vi "AD5535 Manager.vi"() -> ()   [LabVIEW 2016]
uses:
  Typedef/AD5535 - Multi sweep settings.ctl
  Typedef/AD5535 - Square wave settings.ctl
  Typedef/AD5535 - States.ctl
  Typedef/AD5535 - Sweep settings.ctl
panel:
  in  "Exit":bool
  in  "Tab Control":T1(tab)
  in  "Reset all to 0":bool
  in  "Update all":bool
  in  "Update channel":bool
  in  "Channel":u8 max=31 step=1
  in  "Value":sgl min=0 max=204.8 step=0.0125 format="%#_g V"
  in  "Vstep":sgl=0.0125 min=0.0125 max=204.8 step=0.0125 format="%#_g V"
  in  "Vstop":sgl min=0 max=204.8 step=0.0125 format="%#_g V"
  in  "Vstart":sgl min=0 max=204.8 step=0.0125 format="%#_g V"
  in  "Channel to sweep":u8 max=31 step=1
  in  "All other chans value":sgl min=0 max=204.8 step=0.0125 format="%#_g V"
  in  "Time interval - Single sweep":u32=10 caption="Time interval" min=10 max=20000 step=5 format="%.0f ms"
  in  "Sweep channel":bool
  in  "Multi-sweep settings":T2 {"Vstep" min=0.0125 max=204.8 step=0.0125 format="%#_g V"; "Vstop" min=0 max=204.8 step=0.0125 format="%#_g V"; "Vstart" min=0 max=204.8 step=0.0125 format="%#_g V"; "Channel to sweep" max=31 step=1}
  in  "Time interval - Multisweep":u32=10 caption="Time interval" min=10 max=20000 step=5 format="%.0f ms"
  in  "Multi-sweep":bool
  in  "Square wave":bool
  in  "Square wave settings":T3={"Square Chan"=0, "Low Value"=0.0, "High Value"=0.0, "Frequency"=0.5, "Duty Cycle"=50} {"Duty Cycle" min=1 max=99 step=1 format="%#_g %%"; "Frequency" min=0.5 max=500.0 step=0.5 format="%#_g Hz"; "High Value" min=0 max=204.8 step=0.0125 format="%#_g V"; "Low Value" min=0 max=204.8 step=0.0125 format="%#_g V"; "Square Chan" max=31 step=1}
  in  "Arduino COM port":refnum<visa-resource-name>
  out "Status":bool
  in  "Connect":bool
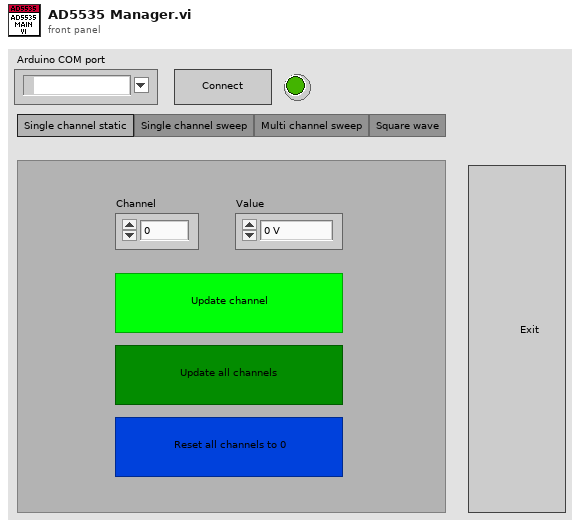
[diagram p1: front panel]
types:
  T1 = enum32{"Single channel static", "Single channel sweep", "Multi channel sweep", "Square wave"}
  T2 = typedef "AD5535 - Multi sweep settings.ctl" = cluster{"Channel to sweep":u8, "Vstart":sgl, "Vstop":sgl, "Vstep":sgl}[]
  T3 = typedef "AD5535 - Square wave settings.ctl" = cluster{"Square Chan":u8, "Low Value":sgl, "High Value":sgl, "Frequency":dbl, "Duty Cycle":u8}
  T4 = typedef "AD5535 - States.ctl" = enum16{"Idle", "Connect", "Update chan", "Update all chan", "Reset all chan", "Sweep channel", "Multi sweep", "Stop sweep", "Square wave", "Exit"}
  T5 = typedef "AD5535 - Sweep settings.ctl" = cluster{"Channel to sweep":u8, "Vstart":sgl, "Vstop":sgl, "Vstep":sgl, "Time interval":u32, "All other chans value":sgl}
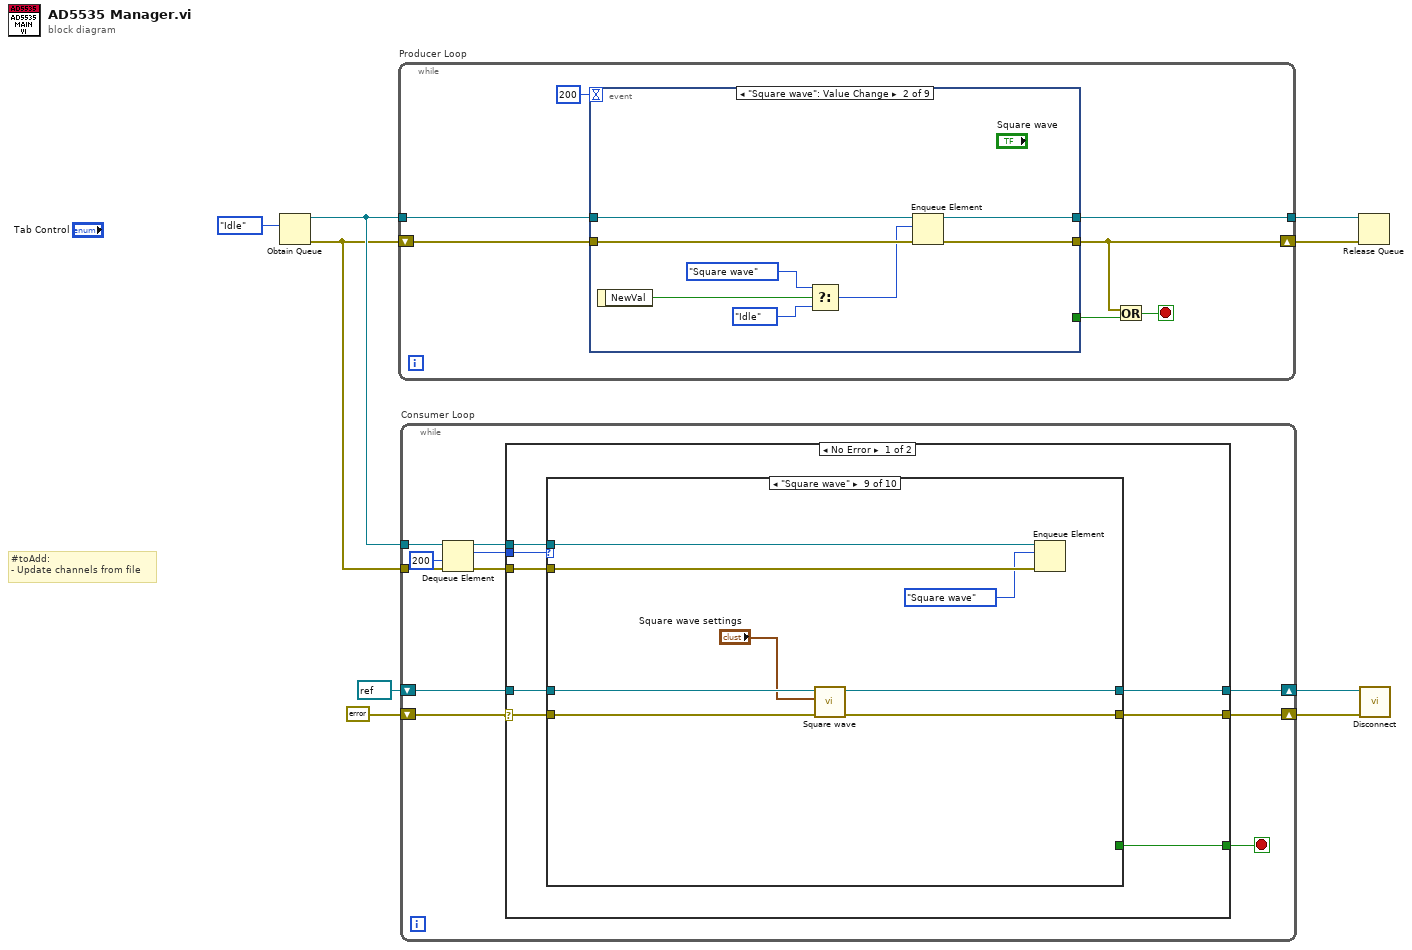
[diagram p0: block diagram]
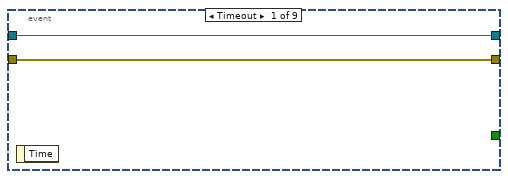
[diagram p2: hidden frame]
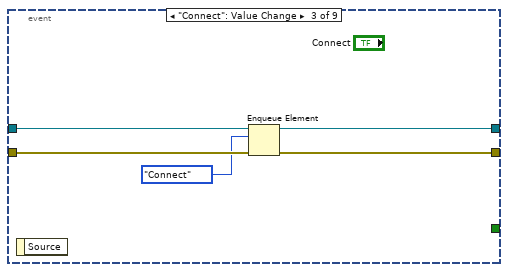
[diagram p3: hidden frame]
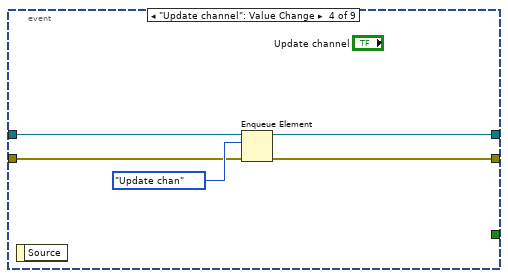
[diagram p4: hidden frame]
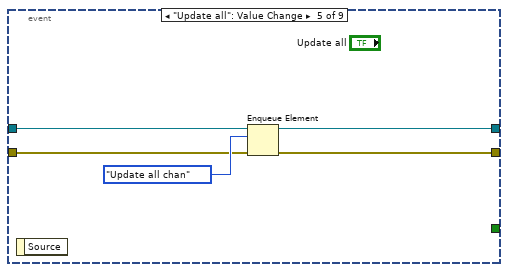
[diagram p5: hidden frame]
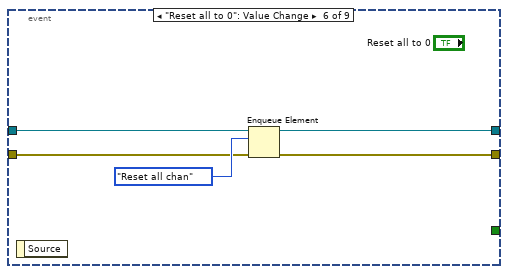
[diagram p6: hidden frame]
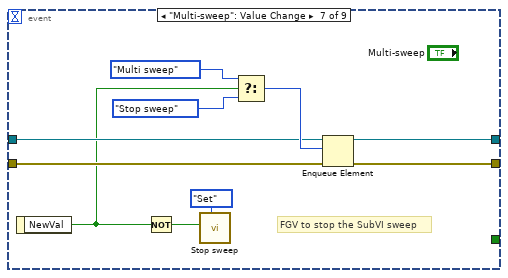
[diagram p7: hidden frame]
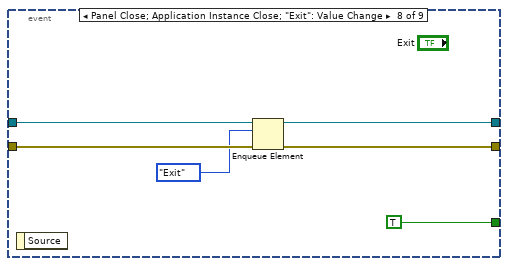
[diagram p8: hidden frame]
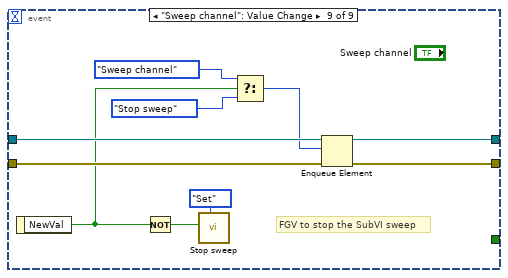
[diagram p9: hidden frame]
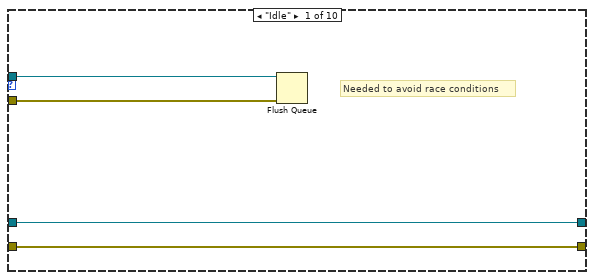
[diagram p10: hidden frame]
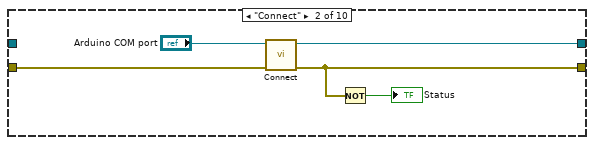
[diagram p11: hidden frame]
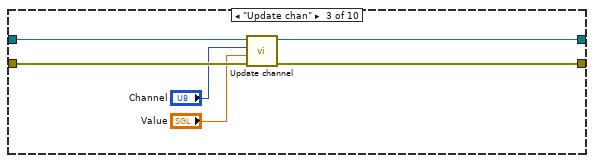
[diagram p12: hidden frame]
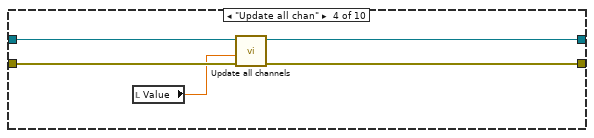
[diagram p13: hidden frame]
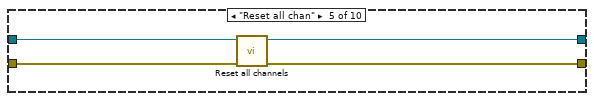
[diagram p14: hidden frame]
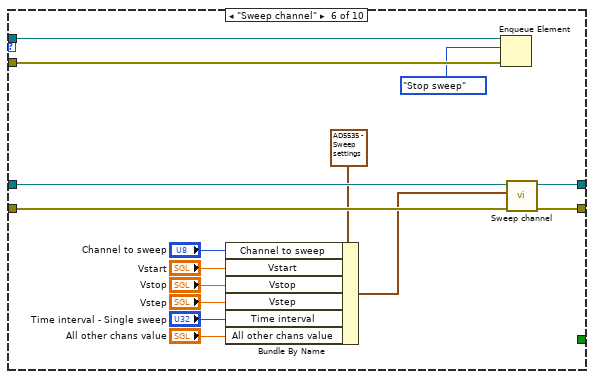
[diagram p15: hidden frame]
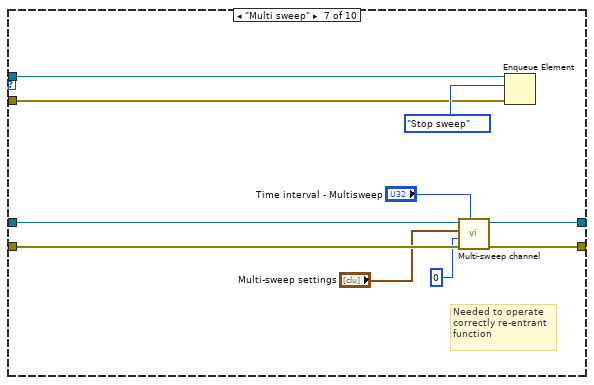
[diagram p16: hidden frame]
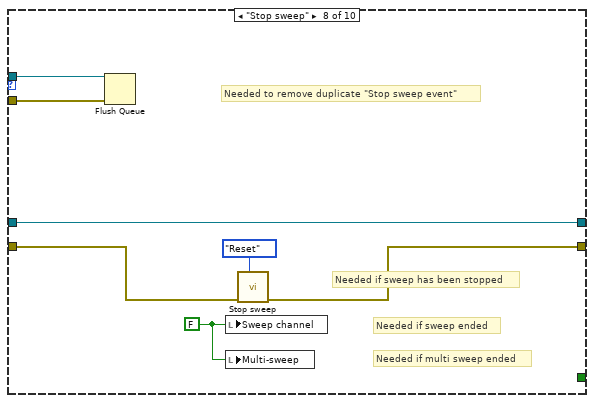
[diagram p17: hidden frame]
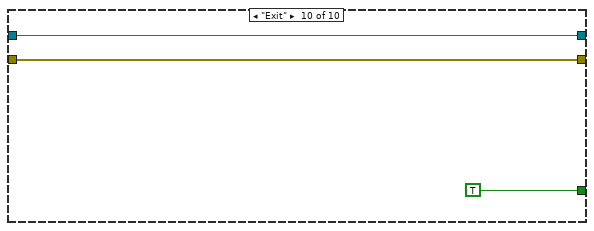
[diagram p18: hidden frame]
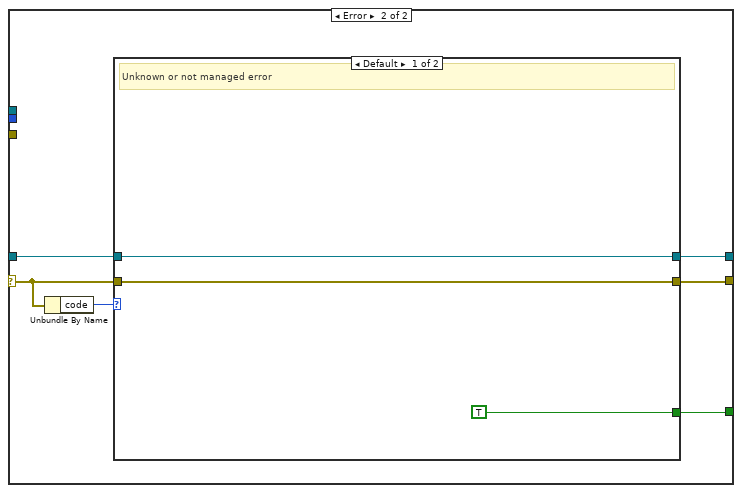
[diagram p19: hidden frame]
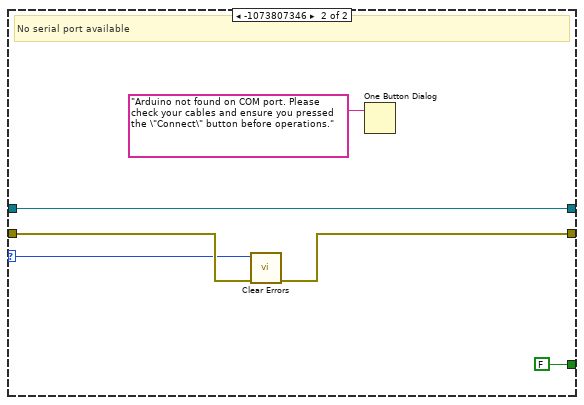
[diagram p20: hidden frame]
diagram:
  # "#toAdd: \n- Update channels from file"
  n1 = Obtain Queue(element data type=AD5535_-_States."Idle") -> (queue out=w6:refnum<queue>, error out=w5:errorcluster)  [unwired: 4 in, 1 out]
  n2 = while "Producer Loop" {
    tunnel: w6 -> [w16]
    shift-right: [w12] -> w7
    shift-left: w5 -> [w15]
    tunnel: [w14] -> w8
    stop <- w13 stop-if-true
    n3 = event shown="[1] \"Square wave\": Value Change" {
      selector: _ -> [_ _ _ _ _ _ _ _ _]
      dyn-events: _ -> [_ _ _ _ _ _ _ _ _]
      timeout: 200 -> [_ _ _ _ _ _ _ _ _]
      tunnel: w16 -> [w18 w26 w31 w35 w40 w45 w51 w62 w72]
      tunnel: [w18 w23 w30 w32 w37 w42 w48 w59 w69] -> w14
      tunnel: w15 -> [w17 w25 w29 w34 w39 w44 w50 w61 w71]
      tunnel: [w17 w24 w28 w33 w38 w43 w49 w60 w70] -> w12
      tunnel: [_ _ _ _ _ _ _ TRUE _] -> w11
      event Timeout {
        n4 = event-data() -> ()  [unwired: 1 in, 1 out]
      }
      event "Square wave": Value Change {
        n5 = event-data() -> ("NewVal"=w22:bool)  [unwired: 1 in]
        n6 = Select(t=AD5535_-_States."Square wave" ("element"), s=w22, f=AD5535_-_States."Idle") -> (s? t:f=w20:T4)
        n7 = Enqueue Element(queue=w26, element=w20, error in (no error)=w25) -> (queue out=w23:refnum<queue>, error out=w24:errorcluster)  [unwired: 1 in, 1 out]
      }
      event "Connect": Value Change {
        n8 = event-data() -> ()  [unwired: 1 in, 1 out]
        n9 = Enqueue Element(queue=w31, element=AD5535_-_States."Connect", error in (no error)=w29) -> (queue out=w30:refnum<queue>, error out=w28:errorcluster)  [unwired: 1 in, 1 out]
      }
      event "Update channel": Value Change {
        n10 = event-data() -> ()  [unwired: 1 in, 1 out]
        n11 = Enqueue Element(queue=w35, element=AD5535_-_States."Update chan", error in (no error)=w34) -> (queue out=w32:refnum<queue>, error out=w33:errorcluster)  [unwired: 1 in, 1 out]
      }
      event "Update all": Value Change {
        n12 = event-data() -> ()  [unwired: 1 in, 1 out]
        n13 = Enqueue Element(queue=w40, element=AD5535_-_States."Update all chan", error in (no error)=w39) -> (queue out=w37:refnum<queue>, error out=w38:errorcluster)  [unwired: 1 in, 1 out]
      }
      event "Reset all to 0": Value Change {
        n14 = event-data() -> ()  [unwired: 1 in, 1 out]
        n15 = Enqueue Element(queue=w45, element=AD5535_-_States."Reset all chan", error in (no error)=w44) -> (queue out=w42:refnum<queue>, error out=w43:errorcluster)  [unwired: 1 in, 1 out]
      }
      event "Multi-sweep": Value Change {
        # "FGV to stop the SubVI sweep"
        n16 = event-data() -> ("NewVal"=w47:bool)  [unwired: 1 in]
        n17 = Not(x=w47) -> (.not. x?=w52:bool)
        n18 = call "Stop sweep.vi"("Status"=enum16{"Set", "Get", "Reset"}."Set", "Exit?"=w52) -> ()  [unwired: 8 in, 2 out]
        n19 = Select(t=AD5535_-_States."Multi sweep" ("element"), s=w47, f=AD5535_-_States."Stop sweep" ("element")) -> (s? t:f=w54:T4)
        n20 = Enqueue Element(queue=w51, element=w54, error in (no error)=w50) -> (queue out=w48:refnum<queue>, error out=w49:errorcluster)  [unwired: 1 in, 1 out]
      }
      event Panel Close; Application Instance Close; "Exit": Value Change {
        n21 = event-data() -> ()  [unwired: 1 in, 1 out]
        n22 = Enqueue Element(queue=w62, element=AD5535_-_States."Exit", error in (no error)=w61) -> (queue out=w59:refnum<queue>, error out=w60:errorcluster)  [unwired: 1 in, 1 out]
      }
      event "Sweep channel": Value Change {
        # "FGV to stop the SubVI sweep"
        n23 = event-data() -> ("NewVal"=w63:bool)  [unwired: 1 in]
        n24 = Not(x=w63) -> (.not. x?=w64:bool)
        n25 = call "Stop sweep.vi"("Status"=enum16{"Set", "Get", "Reset"}."Set", "Exit?"=w64) -> ()  [unwired: 8 in, 2 out]
        n26 = Select(t=AD5535_-_States."Sweep channel" ("element"), s=w63, f=AD5535_-_States."Stop sweep" ("element")) -> (s? t:f=w66:T4)
        n27 = Enqueue Element(queue=w72, element=w66, error in (no error)=w71) -> (queue out=w69:refnum<queue>, error out=w70:errorcluster)  [unwired: 1 in, 1 out]
      }
    }
    n28 = Or(x=w12, y=w11) -> (x .or. y?=w13:bool)
  }
  n29 = while "Consumer Loop" {
    tunnel: w6 -> [w83]
    tunnel: w5 -> [w82]
    shift-right: [w79] -> w2
    shift-left: errorcluster {"status"=FALSE, "code"=0, "source"=""} ("error out") -> [w76]
    shift-right: [w78] -> w3
    shift-left: refnum<visa-resource-name> refnum ("Arduino Port out") -> [w77]
    stop <- w80 stop-if-true
    n30 = Dequeue Element(queue=w83, timeout in ms (-1)=200, error in (no error)=w82) -> (queue out=w75:refnum<queue>, element=w81:T4, error out=w74:errorcluster)  [unwired: 1 out]
    n31 = case shown="No Error" w76 {
      selector: w76 -> [w86 w160]
      tunnel: w81 -> [w91 _]
      tunnel: [w90 w161] -> w80
      tunnel: [w89 w159] -> w79
      tunnel: [w88 w162] -> w78
      tunnel: w77 -> [w87 w163]
      tunnel: w75 -> [w85 _]
      tunnel: w74 -> [w84 _]
      frame No Error {
        n32 = case shown="\"Square wave\"" w91 {
          tunnel: [_ _ _ _ _ _ _ _ _ TRUE] -> w90
          tunnel: [w94 w97 w103 w108 w113 w128 w136 w144 w153 w157] -> w89
          tunnel: w86 -> [w94 w99 w104 w109 w114 w129 w134 w145 w154 w157]
          tunnel: [w95 w98 w105 w110 w112 w127 w137 w147 w152 w156] -> w88
          tunnel: w87 -> [w95 _ w106 w111 w115 w130 w135 w147 w155 w156]
          tunnel: w85 -> [w93 _ _ _ _ w118 w139 w143 w151 _]
          tunnel: w84 -> [w92 _ _ _ _ w117 w138 w142 w150 _]
          frame "Idle" {
            # "Needed to avoid race conditions"
            n33 = Flush Queue(queue=w93, error in (no error)=w92) -> ()  [unwired: 3 out]
          }
          frame "Connect" {
            n34 = call "Connect.vi"("Error In"=w99, "Arduino Port"="Arduino COM port") -> ("Error Out"=w97:errorcluster, "Arduino Port out"=w98:refnum<visa-resource-name>)  [unwired: 8 in]
            n35 = Not(x=w97) -> (.not. x?=→"Status":bool)
          }
          frame "Update chan" {
            n36 = call "Update channel.vi"("Error In"=w104, "Value"="Value", "Channel"="Channel", "Arduino Port"=w106) -> ("Error Out"=w103:errorcluster, "Arduino Port out"=w105:refnum<visa-resource-name>)  [unwired: 6 in]
          }
          frame "Update all chan" {
            n37 = local read "Value"() -> (w107:sgl)
            n38 = call "Update all channels.vi"("Error In"=w109, "Value"=w107, "Arduino Port"=w111) -> ("Error Out"=w108:errorcluster, "Arduino Port out"=w110:refnum<visa-resource-name>)  [unwired: 7 in]
          }
          frame "Reset all chan" {
            n39 = call "Reset all channels.vi"("Error In"=w114, "Arduino Port"=w115) -> ("Error Out"=w113:errorcluster, "Arduino Port out"=w112:refnum<visa-resource-name>)  [unwired: 8 in]
          }
          frame "Sweep channel" {
            n40 = Bundle By Name(cluster=T5 {"Channel to sweep"=0, "Vstart"=0.0, "Vstop"=0.0, "Vstep"=0.0125, "Time interval"=10, "All other chans value"=0.0} ("Sweep settings"), "Channel to sweep"="Channel to sweep", "Vstart"="Vstart", "Vstop"="Vstop", "Vstep"="Vstep", "Time interval"="Time interval - Single sweep", "All other chans value"="All other chans value") -> (w125:T5)
            n41 = Enqueue Element(queue=w118, element=AD5535_-_States."Stop sweep", error in (no error)=w117) -> ()  [unwired: 1 in, 3 out]
            n42 = call "Sweep channel.vi"("Error In"=w129, "Sweep settings"=w125, "Arduino Port"=w130) -> ("Error Out"=w128:errorcluster, "Arduino Port out"=w127:refnum<visa-resource-name>)  [unwired: 7 in]
          }
          frame "Multi sweep" {
            # "Needed to operate\ncorrectly re-entrant\nfunction"
            n43 = call "Multi-sweep channel.vi"("Time interval"="Time interval - Multisweep", "Error In"=w134, "Index"=0, "Multi-sweep settings"="Multi-sweep settings", "Arduino Port"=w135) -> ("Error Out"=w136:errorcluster, "Arduino Port out"=w137:refnum<visa-resource-name>)  [unwired: 5 in]
            n44 = Enqueue Element(queue=w139, element=AD5535_-_States."Stop sweep", error in (no error)=w138) -> ()  [unwired: 1 in, 3 out]
          }
          frame "Stop sweep" {
            w141 = FALSE ("Sweep channel")
            # "Needed if multi sweep ended"
            # "Needed to remove duplicate \"Stop sweep event\""
            # "Needed if sweep has been stopped"
            # "Needed if sweep ended"
            n45 = Flush Queue(queue=w143, error in (no error)=w142) -> ()  [unwired: 3 out]
            n46 = local write "Sweep channel"(w141) -> ()
            n47 = local write "Multi-sweep"(w141) -> ()
            n48 = call "Stop sweep.vi"("Status"=enum16{"Set", "Get", "Reset"}."Reset", "Error In"=w145) -> ("Error Out"=w144:errorcluster)  [unwired: 8 in, 1 out]
          }
          frame "Square wave" {
            n49 = call "Square wave.vi"("Error In"=w154, "Square wave settings"="Square wave settings", "Arduino Port"=w155) -> ("Error Out"=w153:errorcluster, "Arduino Port out"=w152:refnum<visa-resource-name>)  [unwired: 7 in]
            n50 = Enqueue Element(queue=w151, element=AD5535_-_States."Square wave", error in (no error)=w150) -> ()  [unwired: 1 in, 3 out]
          }
          frame "Exit" {
          }
        }
      }
      frame Error {
        # "Error management"
        n51 = Unbundle By Name(w160) -> ("code"=w164:i32)
        n52 = case shown="Default" w164 {
          selector: w164 -> [_ w169]
          tunnel: [w167 w173] -> w162
          tunnel: w163 -> [w167 w173]
          tunnel: [TRUE FALSE] -> w161
          tunnel: [w165 w170] -> w159
          tunnel: w160 -> [w165 w171]
          frame Default {
            # "Unknown or not managed error"
          }
          frame -1073807346 {
            # "No serial port available"
            n53 = call <vilib>:"Clear Errors.vi"("error in (no error)"=w171, "specific error code to clear (0: all)"=w169) -> ("error out"=w170:errorcluster)  [unwired: 4 in, 1 out]
            n54 = One Button Dialog(message="Arduino not found on COM port. Please check your cables and ensure you pressed the \"Connect\" button before operations.") -> ()  [unwired: 1 in, 1 out]
          }
        }
      }
    }
  }
  n55 = Release Queue(queue=w8, error in (no error)=w7) -> ()  [unwired: 1 in, 3 out]
  n56 = call "Disconnect.vi"("Error In"=w2, "Arduino Port"=w3) -> ()  [unwired: 9 in, 1 out]
